vi "Set Temperature.vi"(8 "error in (no error)":errorcluster, 9 "Internal?":bool, 10 "Setpoint":dbl, 11 "Lauda Settings":T1) -> (0 "error out":errorcluster, 1 "Connection Error":bool, 3 "Lauda Settings":T1)   [LabVIEW 2018, in "Lauda TCU.lvlib"]
uses:
  Lauda TCU.lvlib
  Lauda Settings.ctl
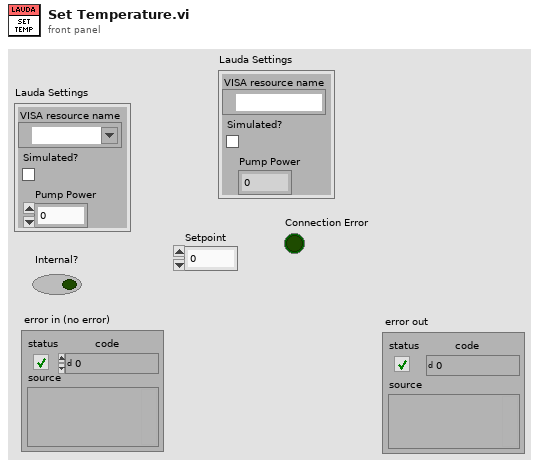
[diagram p1: front panel]
types:
  T1 = typedef "Lauda TCU.lvlib/Lauda Settings.ctl" = cluster{"VISA resource name":refnum<visa-resource-name>, "Simulated?":bool, "Pump Power":i32}
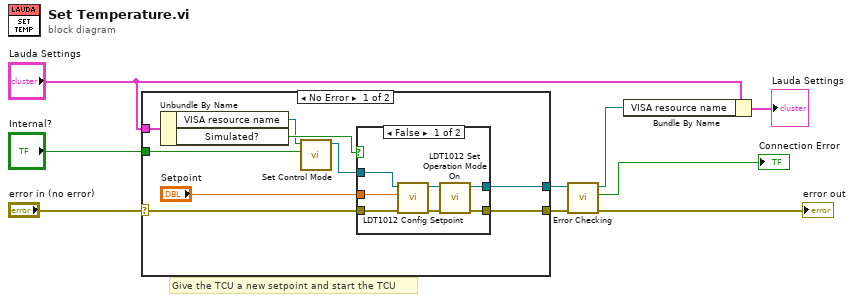
[diagram p0: block diagram]
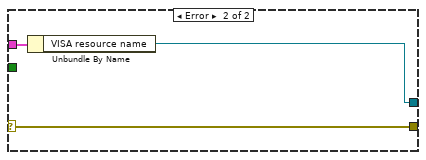
[diagram p3: hidden frame]
diagram:
  # "Give the TCU a new setpoint and start the TCU"
  n1 = case shown="No Error" "error in (no error)" {
    selector: "error in (no error)" -> [w18 w30]
    tunnel: "Lauda Settings" -> [w14 w29]
    tunnel: [w17 w30] -> w7
    tunnel: [w16 w28] -> w8
    tunnel: "Internal?" -> [w12 _]
    frame No Error {
      n2 = Unbundle By Name(w14) -> ("VISA resource name"=w11:refnum<visa-resource-name>, "Simulated?"=w15:bool)
      n3 = call "Set Control Mode.vi"("Internal Control"=w12, "VISA session"=w11) -> ("dup VISA session"=w10:refnum<visa-resource-name>)  [unwired: 8 in, 1 out]
      n4 = case shown="False" w15 {
        tunnel: w18 -> [w23 w27]
        tunnel: [w19 w27] -> w17
        tunnel: [w20 w26] -> w16
        tunnel: w10 -> [w25 w26]
        tunnel: "Setpoint" -> [w24 _]
        frame False {
          n5 = call "LDT1012 Config Setpoint.vi"("error in (no error)"=w23, "Setpoint (20.00 °C: Default)"=w24, "VISA session"=w25) -> ("error out"=w22:errorcluster, "dup VISA session"=w21:refnum<visa-resource-name>)  [unwired: 7 in]
          n6 = call "LDT1012 Set Operation Mode On.vi"("error in (no error)"=w22, "VISA session"=w21) -> ("error out"=w19:errorcluster, "dup VISA session"=w20:refnum<visa-resource-name>)  [unwired: 8 in]
        }
        frame True {
        }
      }
    }
    frame Error {
      n7 = Unbundle By Name(w29) -> ("VISA resource name"=w28:refnum<visa-resource-name>)
    }
  }
  n8 = call "Error Checking.vi"("error in (no error)"=w7, "VISA resource name"=w8) -> ("error out"=→"error out":errorcluster, "Connection Error"=→"Connection Error":bool, "VISA resource name"=w5:refnum<visa-resource-name>)  [unwired: 7 in]
  n9 = Bundle By Name(cluster="Lauda Settings", "VISA resource name"=w5) -> (→"Lauda Settings":T1)
